vi "TCP.vi"() -> (3 "data out":string)   [LabVIEW 2020]
panel:
  out "error out":errorcluster
  in  "Server Closed":string="The server VI closed the connection."
  in  "Stop":bool
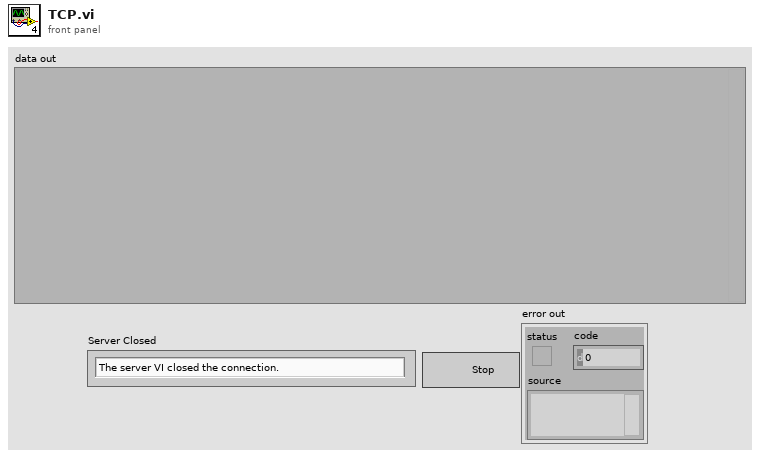
[diagram p1: front panel]
types:
  T1 = enum16{"Standard", "Buffered", "CRLF", "Immediate"}
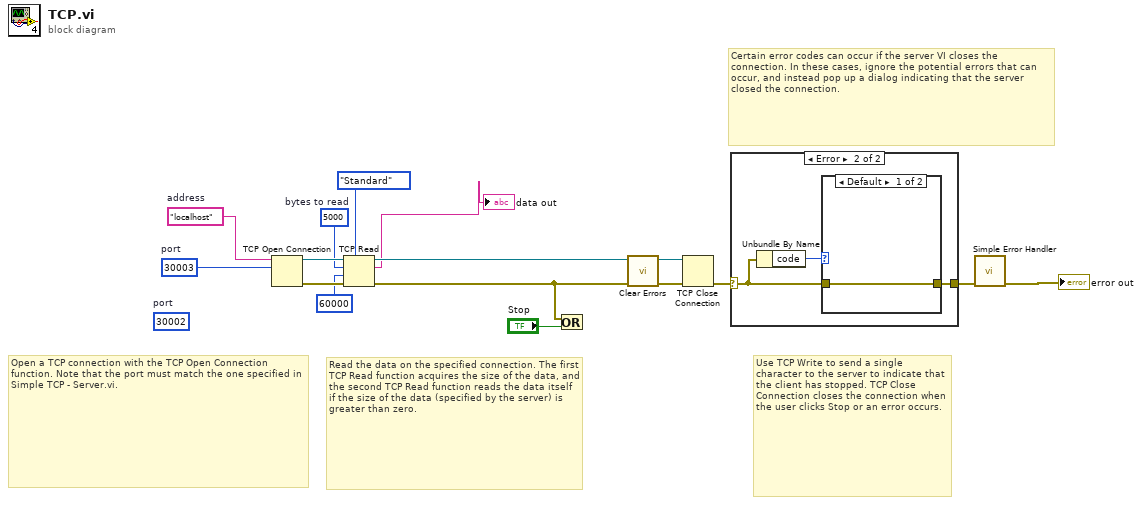
[diagram p0: block diagram]
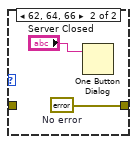
[diagram p3: hidden frame]
diagram:
  w8 = 5000  # bytes to read
  (unwired) u16 30002  # port
  w1 = u16 30003  # port
  w11 = "localhost"  # address
  # "Certain error codes can occur if the server VI closes the connection. In these cases, ignore the potential errors that can occur, and instead pop up a dialog indicating that the server closed the connection."
  # "Use TCP Write to send a single character to the server to indicate that the client has stopped. TCP Close Connection closes the connection when the user clicks Stop or an error occurs."
  # "Read the data on the specified connection. The first TCP Read function acquires the size of the data, and the second TCP Read function reads the data itself if the size of the data (specified by the server) is greater than zero."
  # "Open a TCP connection with the TCP Open Connection function. Note that the port must match the one specified in Simple TCP - Server.vi."
  n1 = TCP Open Connection(address=w11, remote port or service name=w1) -> (connection ID=w15:refnum<k5>, error out=w14:errorcluster)  [unwired: 3 in]
  n2 = TCP Read(connection ID=w15, bytes to read=w8, error in (no error)=w14, 7:T1."Standard" ("mode (standard)"), 9:60000 ("timeout ms (25000)")) -> (connection ID out=w10:refnum<k5>, data out=→"data out":string, error out=w9:errorcluster)
  n3 = Or(x=w9, y="Stop") -> ()  [unwired: 1 out]
  n4 = call <vilib>:"Clear Errors.vi"("error in (no error)"=w9) -> ("error out"=w2:errorcluster)  [unwired: 5 in, 1 out]
  n5 = TCP Close Connection(connection ID=w10, error in (no error)=w2) -> (error out=w13:errorcluster)  [unwired: 1 in, 1 out]
  n6 = case shown="Error" w13 {
    selector: w13 -> [w16 w18]
    tunnel: [w16 w17] -> w12
    frame No Error {
    }
    frame Error {
      n7 = Unbundle By Name(w18) -> ("code"=w19:i32)
      n8 = case shown="Default" w19 {
        tunnel: w18 -> [w20 _]
        tunnel: [w20 w22] -> w17
        frame Default {
        }
        frame 62, 64, 66 {
          w22 = errorcluster {"status"=FALSE, "code"=0, "source"=""}  # No error
          n9 = One Button Dialog(message="Server Closed") -> ()  [unwired: 1 in, 1 out]
        }
      }
    }
  }
  n10 = call <vilib>:"Simple Error Handler.vi"("error in (no error)"=w12) -> ("error out"=→"error out":errorcluster)  [unwired: 4 in, 4 out]
